vi "Write Function Name.vi"(8 "error in (no error)":errorcluster, 10 "Function Name":string, 11 "Tell Controller to Check Fcn and Dev Selection Msg in":refnum<class "Tell Controller to Check Fcn and Dev Selection Msg.lvclass">) -> (0 "error out":errorcluster, 3 "Tell Controller to Check Fcn and Dev Selection Msg out":refnum<class "Tell Controller to Check Fcn and Dev Selection Msg.lvclass">)   [LabVIEW 2016, in "Controller UI.lvlib" / "Tell Controller to Check Fcn and Dev Selection Msg.lvclass"]
uses:
  <userlib>/Common Components/Controller UI Messages/Tell Controller to Check Fcn and Dev Selection Msg/Tell Controller to Check Fcn and Dev Selection Msg.lvclass
  <userlib>/Common Components/Controller UI Messages/Tell Controller to Check Fcn and Dev Selection Msg/Tell Controller to Check Fcn and Dev Selection Msg.lvclass/Tell Controller to Check Fcn and Dev Selection Msg.ctl
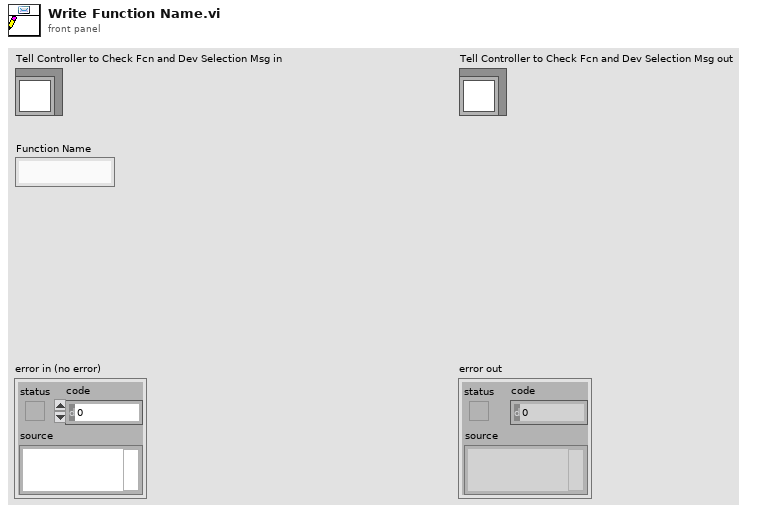
[diagram p1: front panel]
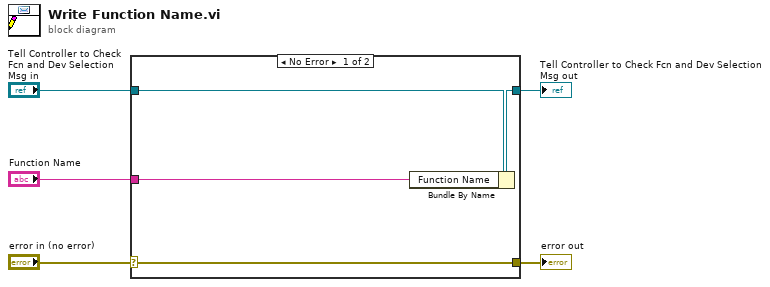
[diagram p0: block diagram]
diagram:
  n1 = case shown="No Error" "error in (no error)" {
    selector: "error in (no error)" -> [w9 w10]
    tunnel: [w9 w10] -> w4
    tunnel: [w7 w11] -> w2
    tunnel: "Tell Controller to Check Fcn and Dev Selection Msg in" -> [w8 w11]
    tunnel: "Function Name" -> [w6 _]
    frame No Error {
      n2 = Bundle By Name(cluster=w8, "Function Name"=w6) -> (w7:refnum<class "Tell Controller to Check Fcn and Dev Selection Msg.lvclass">)
    }
    frame Error {
    }
  }
  "error out" <- w4
  "Tell Controller to Check Fcn and Dev Selection Msg out" <- w2
